vi "SetIndividualJoints.vi"(0 "Mode":enum16{"Position", "Velocity", "Effort"}(ring)=enum."Velocity", 1 "node":string, 2 "Joint States":T1(array[cluster]), 3 "error in":errorcluster) -> (6 "error out":errorcluster)   [LabVIEW 2013]
uses:
  ROS/Code/SubVIs/BaxterSide.ctl
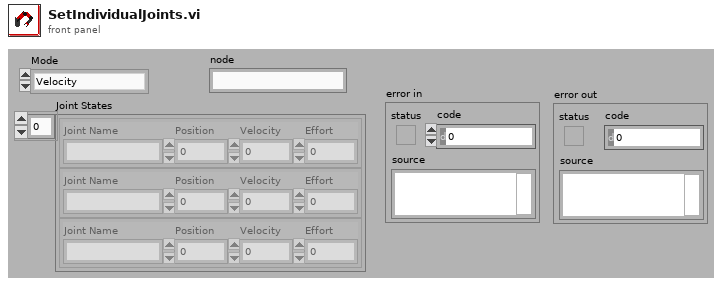
[diagram p1: front panel]
types:
  T1 = cluster{"Joint Name":string, "Position":dbl, "Velocity":dbl, "Effort":dbl}[]
  T2 = typedef "BaxterSide.ctl" = enum16{"left", "right"}
  T3 = typedef "_ROSControl.ctl" = cluster{"topic port":u16, "Node":string, "topic":string, "type":string, "node port":u32, "error ":errorcluster, "Direction":T4, "APIs":string[]}
  T4 = typedef "_ROSDirection.ctl" = enum16{"Node", "Publisher", "Subscriber", "Service Client"}
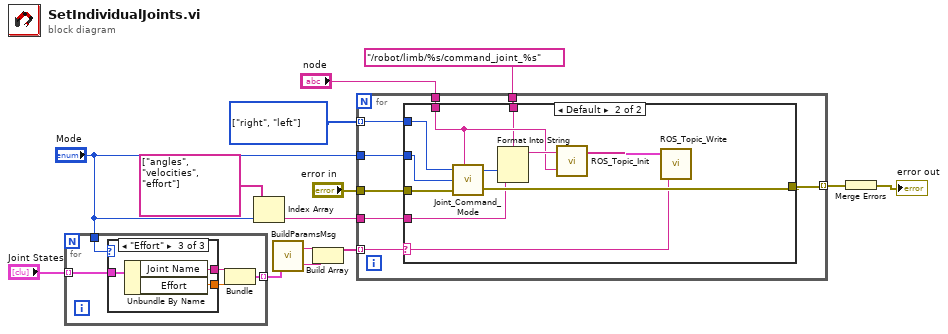
[diagram p0: block diagram]
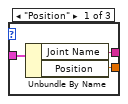
[diagram p2: hidden frame]
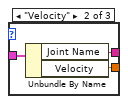
[diagram p3: hidden frame]
diagram:
  w12 = T2[] [enum."right", enum."left"] items=["left", "right"]
  n1 = for {
    tunnel: "Joint States" -> [w19] mode=indexing
    tunnel: "Mode" -> [w18]
    tunnel: [w15] -> w1 mode=indexing
    n2 = case shown="\"Effort\"" w18 {
      tunnel: w19 -> [w22 w25 w28]
      tunnel: [w21 w24 w27] -> w17
      tunnel: [w20 w23 w26] -> w16
      frame "Position" {
        n3 = Unbundle By Name(w22) -> ("Joint Name"=w21:string, "Position"=w20:dbl)
      }
      frame "Velocity" {
        n4 = Unbundle By Name(w25) -> ("Joint Name"=w24:string, "Velocity"=w23:dbl)
      }
      frame "Effort" {
        n5 = Unbundle By Name(w28) -> ("Joint Name"=w27:string, "Effort"=w26:dbl)
      }
    }
    n6 = Bundle("Joint Name"=w17, "Effort"=w16) -> (w15:cluster{"Joint Name":string, "Effort":dbl})  [unwired: 1 in]
  }
  n7 = Index Array(array=string[] ["angles", "velocities", "effort"], index="Mode") -> (element=w4:string)
  n8 = call "BuildParamsMsg.vi"("Parameters"=w1) -> ("left msg"=w8:string, "right msg"=w9:string)
  n9 = Build Array(w9, w8) -> (w7:string[])
  n10 = for {
    tunnel: [w36] -> w10 mode=indexing
    tunnel: "error in" -> [w35]
    tunnel: "node" -> [w33]
    tunnel: w12 -> [w34] mode=indexing
    tunnel: "Mode" -> [w32]
    tunnel: w7 -> [w31] mode=indexing
    tunnel: "/robot/limb/%s/command_joint_%s" ("topic") -> [w30]
    tunnel: w4 -> [w29]
    n11 = case shown="Default" w31 {
      selector: w31 -> [_ w43]
      tunnel: [w37 w44] -> w36
      tunnel: w35 -> [w37 w47]
      tunnel: w34 -> [_ w42]
      tunnel: w33 -> [_ w41]
      tunnel: w32 -> [_ w38]
      tunnel: w30 -> [_ w40]
      tunnel: w29 -> [_ w39]
      frame "" {
      }
      frame Default {
        n12 = call "Joint_Command_Mode.vi"("Side"=w42, "node"=w41, "Mode"=w38, "error in"=w47) -> ("error out"=w44:errorcluster)  [unwired: 2 in]
        n13 = Format Into String(format string=w40, w42, w39) -> (resulting string=w46:string)  [unwired: 2 in, 1 out]
        n14 = call "ROS_Topic_Init.vi"("node"=w41, "topic"=w46) -> ("ROS out"=w45:T3)  [unwired: 1 in]
        n15 = call "ROS_Topic_Write.vi"("Msg in"=w43, "ROS in"=w45) -> ()  [unwired: 2 in, 1 out]
      }
    }
  }
  n16 = Merge Errors(w10) -> (→"error out":errorcluster)
